vi "Directory CRC Validation.vi"(8 "error in (no error)":errorcluster, 11 "Folder Path":path) -> (0 "error out":errorcluster, 3 "CRC32 Value":u32)   [LabVIEW 2018]
doc: "A short LabVIEW routine to calculate the CRC32 value on one (or more) files. Uses the same algorithm as WinZip and Microsoft's CRC305 application. Written entirely in LabVIEW, this routine calculates a 32-bit CRC value of an entire file (text or binary)."
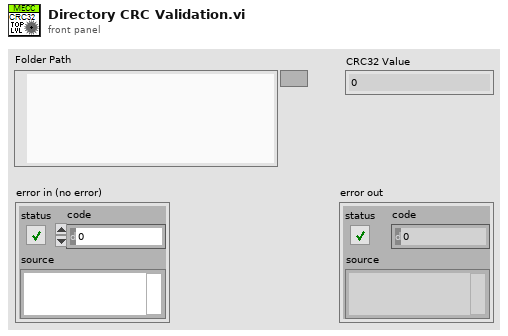
[diagram p1: front panel]
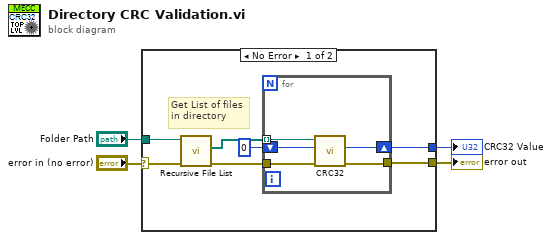
[diagram p0: block diagram]
diagram:
  n1 = case shown="No Error" "error in (no error)" {
    selector: "error in (no error)" -> [w5 w17]
    tunnel: "Folder Path" -> [w11 _]
    tunnel: [w9 _] -> w3
    tunnel: [w6 w17] -> w2
    frame No Error {
      # "Get List of files\nin directory"
      n2 = call <vilib>:"Recursive File List.vi"("error in (no error)"=w5, "Folder Path"=w11) -> ("error out"=w7:errorcluster, "All Files in Dir"=w10:path[])  [unwired: 5 in, 3 out]
      n3 = for {
        tunnel: w10 -> [w16] mode=indexing
        shift-right: [w14] -> w9
        shift-left: u32 0 ("CRC32Value") -> [w15]
        tunnel: w7 -> [w13]
        tunnel: [w12] -> w6
        n4 = call "CRC32.vi"("error in (no error)"=w13, "CRCBuffer"=w15, "FileToCalculate"=w16) -> ("error out"=w12:errorcluster, "CRC32Value"=w14:u32)  [unwired: 7 in]
      }
    }
    frame Error {
    }
  }
  "CRC32 Value" <- w3
  "error out" <- w2
